vi "VGF Time.vi"(10 "Enum":enum16{"Set Time", "Elapsed Time"}(ring), 11 "Time tarjet":i32) -> (3 "Time lapsed":bool)   [LabVIEW 2019, in "Analisis.lvlib"]
doc: "FGV dedicated to analize the time stablished by suser to storage the data obtained in a data base"
uses:
  Analisis.lvlib
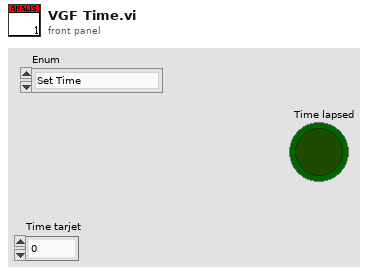
[diagram p1: front panel]
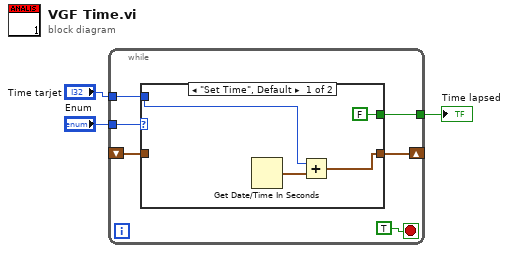
[diagram p0: block diagram]
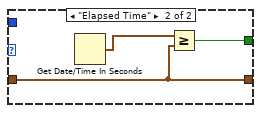
[diagram p2: hidden frame]
diagram:
  n1 = while {
    shift-right: [w8] -> _
    shift-left: _ -> [w7]
    tunnel: "Enum" -> [w9]
    tunnel: [w5] -> w2
    tunnel: "Time tarjet" -> [w4]
    stop <- TRUE stop-if-true
    n2 = case shown="\"Set Time\", Default" w9 {
      tunnel: [w12 w14] -> w8
      tunnel: w7 -> [_ w14]
      tunnel: [FALSE w16] -> w5
      tunnel: w4 -> [w11 _]
      frame "Set Time", Default {
        n3 = Get Date/Time In Seconds() -> (seconds since 1Jan1904=w13:timestamp)
        n4 = Add(x=w11, y=w13) -> (x+y=w12:timestamp)
      }
      frame "Elapsed Time" {
        n5 = Get Date/Time In Seconds() -> (seconds since 1Jan1904=w15:timestamp)
        n6 = Greater Or Equal?(x=w15, y=w14) -> (x >= y?=w16:bool)
      }
    }
  }
  "Time lapsed" <- w2
